vi "[C] Log To File.vi"() -> ()   [LabVIEW 2014]
uses:
  <userlib>/_OpenG.lib/file/file.llb/Build Path - Traditional__ogtk.vi
  Sensor Reading.ctl
panel:
  in  "Database File":path=path "C:/Users/Chris/Sync/Tower Snippets/Users/Chris/Downloads/Tower Snippets/New Model/database.txt"
  in  "Message Q":refnum<queue>
  in  "Data Q":refnum<queue>
  in  "Sensor Reading":T1
  # "INPUT PARAMETERS"
  # "INTERNAL VARIABLES - could possibly be set programatically..."
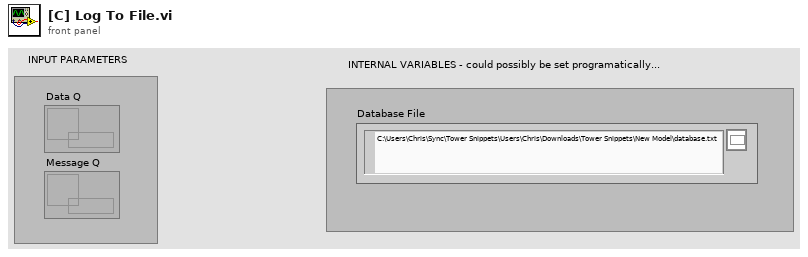
[diagram p1: front panel]
types:
  T1 = typedef "Sensor Reading.ctl" = cluster{"Sensor Name":string, "Timestamp":string, "Data Chunk":string}
  T2 = enum16{"open", "replace", "create", "open or create", "replace or create", "replace or create with confirmation"}
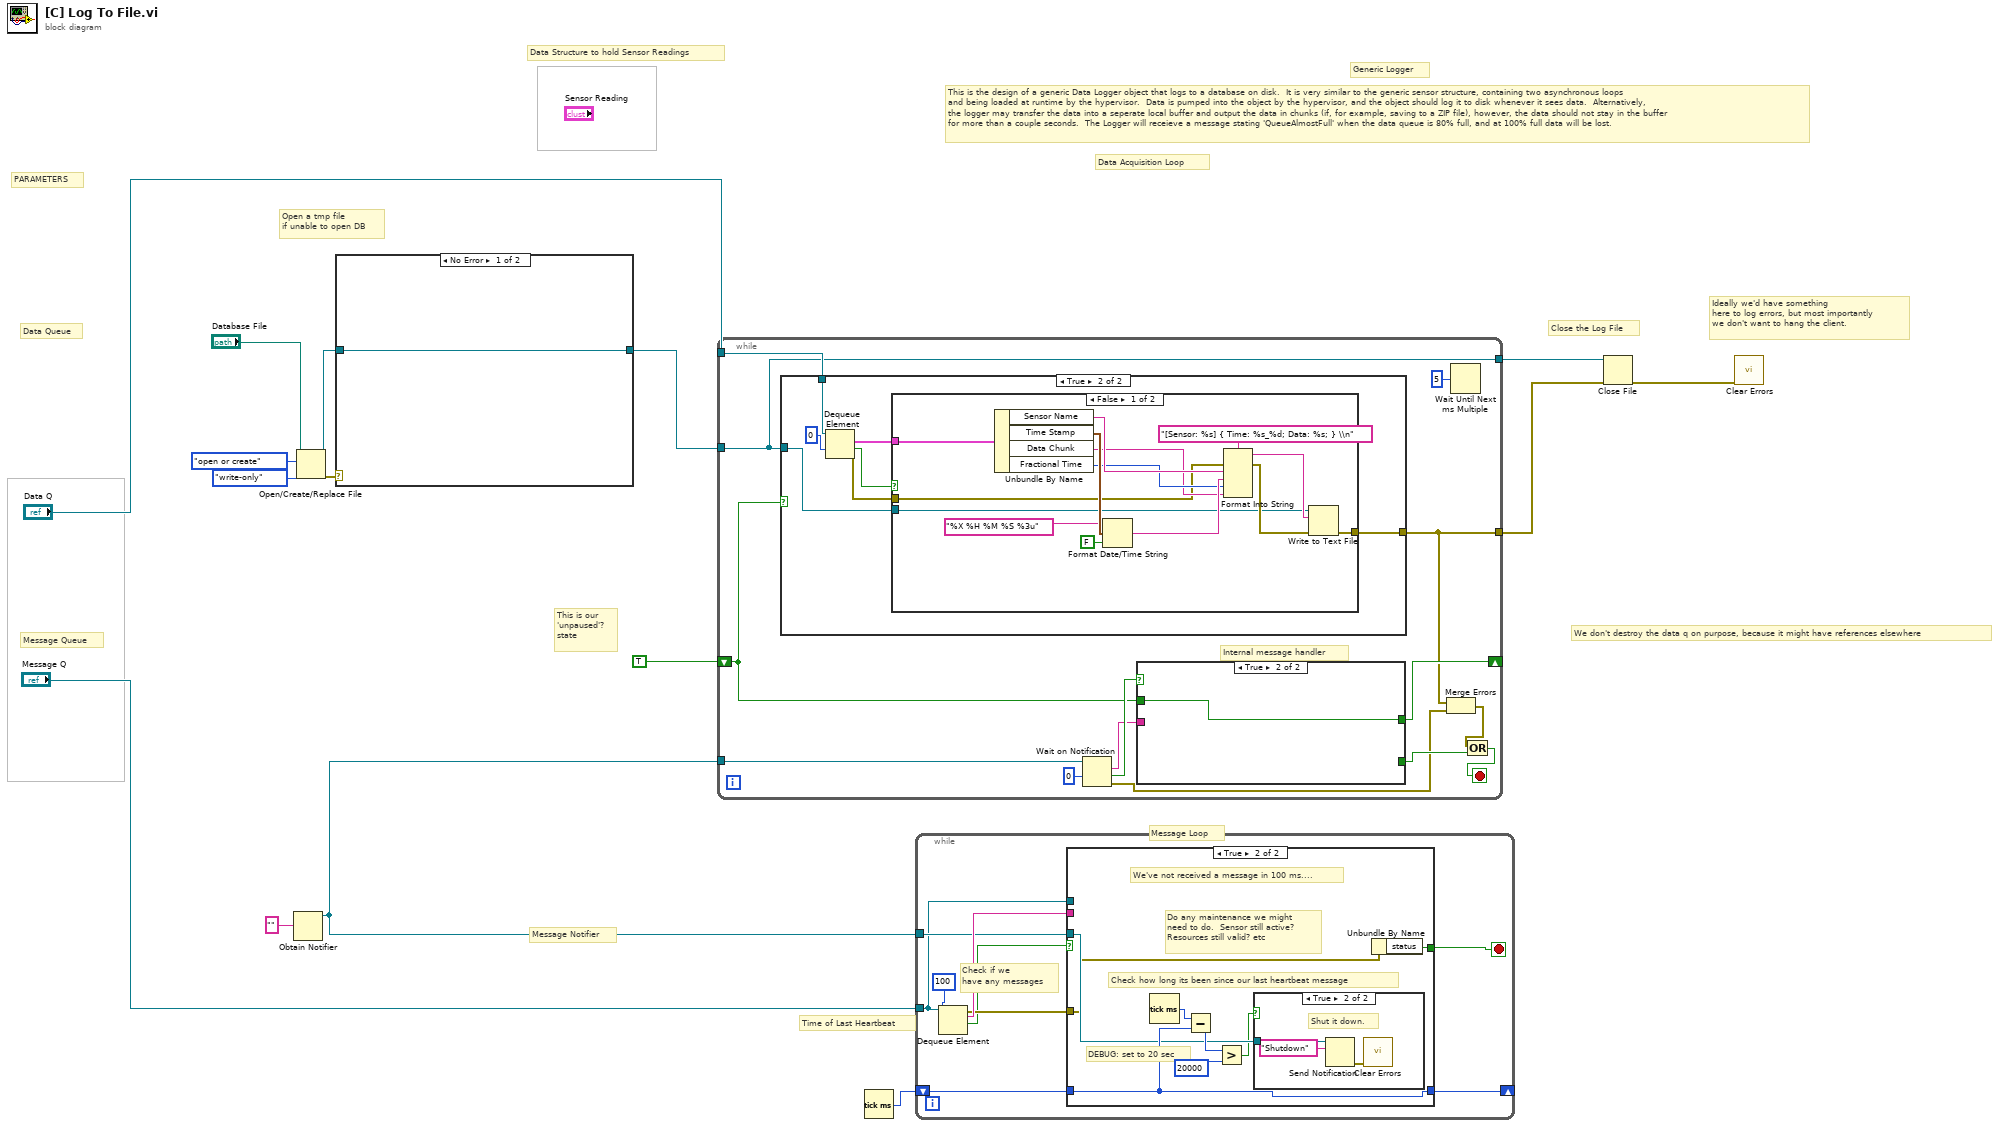
[diagram p0: block diagram]
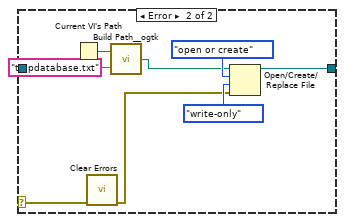
[diagram p2: hidden frame]
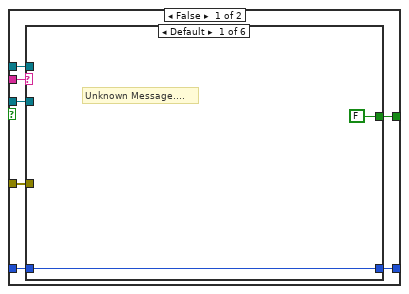
[diagram p3: hidden frame]
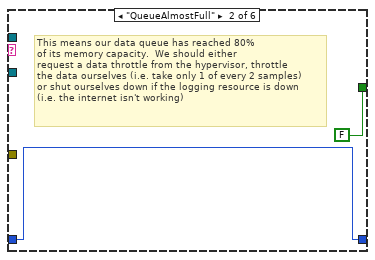
[diagram p4: hidden frame]
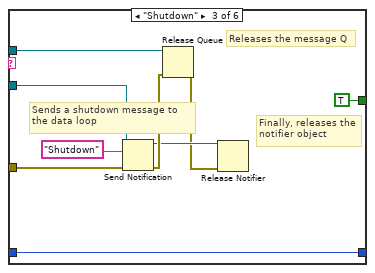
[diagram p5: hidden frame]
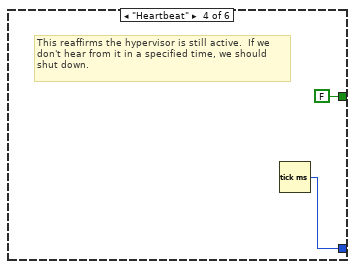
[diagram p6: hidden frame]
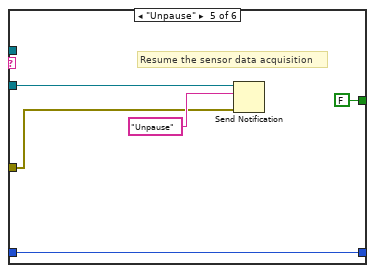
[diagram p7: hidden frame]
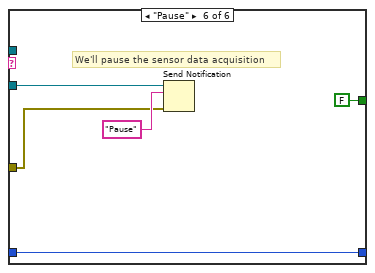
[diagram p8: hidden frame]
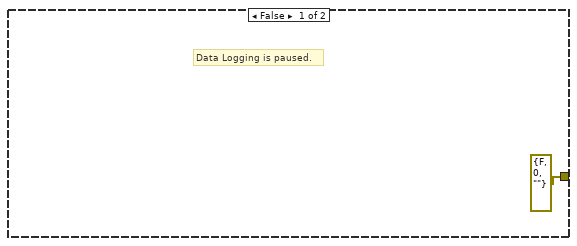
[diagram p10: hidden frame]
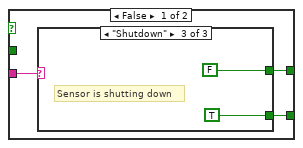
[diagram p12: hidden frame]
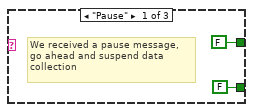
[diagram p13: hidden frame]
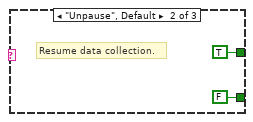
[diagram p14: hidden frame]
diagram:
  # "Ideally we'd have something \nhere to log errors, but most importantly\nwe don't want to hang the client."
  # "Time of Last Heartbeat"
  # "Close the Log File"
  # "Open a tmp file\nif unable to open DB"
  # "This is the design of a generic Data Logger object that logs to a database on disk.  It is very similar to the generic sensor structure, containing two asynchronous loops\nand being loaded at runtime by the hypervisor.  Data is pumped into the object by the hypervisor, and the object should log it to disk whenever it sees data.  Alternatively,\nthe logger may transfer the data into a seperate local buffer and output the data in chunks (if, for example, saving to a ZIP file), however, the data should not stay in the buffer\nfor more than a couple seconds.  The Logger will receieve a message stating 'QueueAlmostFull' when the data queue is 80% full, and at 100% full data will be lost."
  # "This is our\n'unpaused'?\nstate"
  # "We don't destroy the data q on purpose, because it might have references elsewhere"
  # "Data Structure to hold Sensor Readings"
  # "Data Acquisition Loop"
  # "Message Loop"
  # "Message Notifier"
  # "Message Queue"
  # "Data Queue"
  # "PARAMETERS"
  # "Generic Logger"
  n1 = Obtain Notifier(notification data type="") -> (notifier out=w15:refnum<notifier>)  [unwired: 3 in, 2 out]
  n2 = Open/Create/Replace File(file path (use dialog)="Database File", operation (0:open)=T2."open or create", access (0:read/write)=enum16{"read/write", "read-only", "write-only"}."write-only") -> (refnum out=w8:refnum<file>, error out=w9:errorcluster)  [unwired: 3 in, 1 out]
  n3 = case shown="No Error" w9 {
    selector: w9 -> [_ w18]
    tunnel: w8 -> [w16 _]
    tunnel: [w16 w22] -> w7
    frame No Error {
    }
    frame Error {
      n4 = Current VI's Path() -> (path=w21:path)
      n5 = call <vilib>:"Clear Errors.vi"("error in (no error)"=w18) -> ("error out"=w17:errorcluster)  [unwired: 5 in, 1 out]
      n6 = call-poly <userlib>:"Build Path__ogtk.vi"("name or relative path"="tmpdatabase.txt", "base path"=w21) -> ("appended path"=w19:path)
      n7 = Open/Create/Replace File(file path (use dialog)=w19, error in=w17, operation (0:open)=T2."open or create", access (0:read/write)=enum16{"read/write", "read-only", "write-only"}."write-only") -> (refnum out=w22:refnum<file>)  [unwired: 2 in, 2 out]
    }
  }
  n8 = while {
    tunnel: "Data Q" -> [w29]
    tunnel: w15 -> [w38]
    shift-right: [w34] -> _
    shift-left: TRUE -> [w33]
    tunnel: w7 -> [w28]
    tunnel: [w28] -> w6
    tunnel: [w27] -> w5
    stop <- w31 stop-if-true
    # "Internal message handler"
    n9 = case shown="True" w33 {
      tunnel: w29 -> [_ w46]
      tunnel: w28 -> [_ w42]
      tunnel: [errorcluster {"status"=FALSE, "code"=0, "source"=""} ("error out") w41] -> w27
      frame False {
        # "Data Logging is paused."
      }
      frame True {
        n10 = Dequeue Element(queue=w46, timeout in ms (-1)=0) -> (element=w43:T1, timed out?=w44:bool, error out=w40:errorcluster)  [unwired: 1 in, 1 out]
        n11 = case shown="False" w44 {
          tunnel: w43 -> [w60 _]
          tunnel: w42 -> [w49 _]
          tunnel: [w48 w61] -> w41
          tunnel: w40 -> [w47 w61]
          frame False {
            n12 = Unbundle By Name(w60) -> ("Sensor Name"=w58:string, "Time Stamp"=w57:timestamp, "Data Chunk"=w53:string, "Fractional Time"=w54:u64)
            n13 = Format Date/Time String(time format string (%c)="%X %H %M %S %3u", seconds (now)=w57, UTC format=FALSE) -> (date/time string=w55:string)
            n14 = Format Into String(format string="[Sensor: %s] { Time: %s_%d; Data: %s; } \\n", error in=w47, w58, w55, w54, w53) -> (resulting string=w50:string, error out=w51:errorcluster)  [unwired: 1 in]
            n15 = Write to Text File(file (use dialog)=w49, text=w50, error in=w51) -> (error out=w48:errorcluster)  [unwired: 1 in, 2 out]
          }
          frame True {
          }
        }
      }
    }
    n16 = Wait on Notification(notifier=w38, timeout in ms (-1)=0) -> (notification=w35:string, timed out?=w36:bool, error out=w26:errorcluster)  [unwired: 2 in, 1 out]
    n17 = case shown="True" w36 {
      tunnel: w35 -> [w64 _]
      tunnel: [w63 _] -> w32
      tunnel: [w62 w71] -> w34
      tunnel: w33 -> [_ w71]
      frame False {
        n18 = case shown="\"Shutdown\"" w64 {
          tunnel: [FALSE FALSE TRUE] -> w63
          tunnel: [FALSE TRUE FALSE] -> w62
          frame "Pause" {
            # "We received a pause message,\ngo ahead and suspend data collection"
          }
          frame "Unpause", Default {
            # "Resume data collection."
          }
          frame "Shutdown" {
            # "Sensor is shutting down"
          }
        }
      }
      frame True {
      }
    }
    n19 = Merge Errors(w27, w26) -> (w25:errorcluster)
    n20 = Wait Until Next ms Multiple(millisecond multiple=u32 5) -> ()  [unwired: 1 out]
    n21 = Or(x=w25, y=w32) -> (x .or. y?=w31:bool)
  }
  n22 = Tick Count (ms)() -> (millisecond timer value=w2:u32)
  n23 = while {
    tunnel: "Message Q" -> [w77]
    tunnel: w15 -> [w78]
    shift-right: [w72] -> _
    shift-left: w2 -> [w73]
    stop <- w79 stop-if-true
    # "Check if we \nhave any messages"
    n24 = Dequeue Element(queue=w77, timeout in ms (-1)=100) -> (element=w80:string, timed out?=w74:bool, error out=w76:errorcluster)  [unwired: 1 in, 1 out]
    n25 = case shown="True" w74 {
      tunnel: w80 -> [w87 _]
      tunnel: [w86 w113] -> w79
      tunnel: w78 -> [w85 w116]
      tunnel: w77 -> [w84 _]
      tunnel: w76 -> [w83 w114]
      tunnel: w73 -> [w82 w117]
      tunnel: [w81 w117] -> w72
      frame False {
        n26 = case shown="Default" w87 {
          tunnel: [FALSE FALSE TRUE FALSE FALSE FALSE] -> w86
          tunnel: w85 -> [_ _ w98 _ w105 w109]
          tunnel: w84 -> [_ _ w99 _ _ _]
          tunnel: w83 -> [_ _ w97 _ w106 w110]
          tunnel: w82 -> [w88 w90 w92 _ w103 w108]
          tunnel: [w88 w90 w92 w102 w103 w108] -> w81
          frame Default {
            # "Unknown Message...."
          }
          frame "QueueAlmostFull" {
            # "This means our data queue has reached 80%\nof its memory capacity.  We should either\nrequest a data throttle from the hypervisor, throttle\nthe data ourselves (i.e. take only 1 of every 2 samples)\nor shut ourselves down if the logging resource is down\n(i.e. the internet isn't working)"
          }
          frame "Shutdown" {
            # "Finally, releases the\nnotifier object"
            # "Releases the message Q"
            # "Sends a shutdown message to \nthe data loop"
            n27 = Send Notification(notification="Shutdown", notifier=w98, error in (no error)=w97) -> (notifier out=w94:refnum<notifier>, error out=w96:errorcluster)
            n28 = Release Queue(queue=w99, error in (no error)=w96) -> (error out=w93:errorcluster)  [unwired: 1 in, 2 out]
            n29 = Release Notifier(notifier=w94, error in (no error)=w93) -> ()  [unwired: 1 in, 3 out]
          }
          frame "Heartbeat" {
            # "This reaffirms the hypervisor is still active.  If we\ndon't hear from it in a specified time, we should\nshut down."
            n30 = Tick Count (ms)() -> (millisecond timer value=w102:u32)
          }
          frame "Unpause" {
            # "Resume the sensor data acquisition"
            n31 = Send Notification(notification="Unpause", notifier=w105, error in (no error)=w106) -> ()  [unwired: 2 out]
          }
          frame "Pause" {
            # "We'll pause the sensor data acquisition"
            n32 = Send Notification(notification="Pause", notifier=w109, error in (no error)=w110) -> ()  [unwired: 2 out]
          }
        }
      }
      frame True {
        # "DEBUG: set to 20 sec"
        # "Check how long its been since our last heartbeat message"
        # "Do any maintenance we might\nneed to do.  Sensor still active?\nResources still valid? etc"
        # "We've not received a message in 100 ms...."
        n33 = Tick Count (ms)() -> (millisecond timer value=w120:u32)
        n34 = Subtract(x=w120, y=w117) -> (x-y=w119:u32)
        n35 = Greater?(x=w119, y=u32 20000) -> (0:w115:bool)
        n36 = case shown="True" w115 {
          tunnel: w116 -> [_ w123]
          frame False {
          }
          frame True {
            # "Shut it down."
            n37 = Send Notification(notification="Shutdown", notifier=w123) -> (error out=w121:errorcluster)  [unwired: 1 in, 1 out]
            n38 = call <vilib>:"Clear Errors.vi"("error in (no error)"=w121) -> ()  [unwired: 5 in, 2 out]
          }
        }
        n39 = Unbundle By Name(w114) -> ("status"=w113:bool)
      }
    }
  }
  n40 = Close File(refnum=w6, error in=w5) -> (error out=w1:errorcluster)  [unwired: 1 out]
  n41 = call <vilib>:"Clear Errors.vi"("error in (no error)"=w1) -> ()  [unwired: 5 in, 2 out]
